vi "Count Up.vi"(7 "Reset":bool, 10 "Increment":bool) -> (2 "Count":i32)   [LabVIEW 2021]
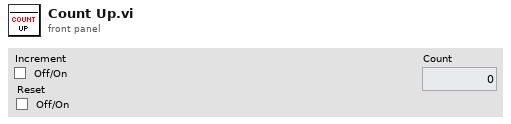
[diagram p1: front panel]
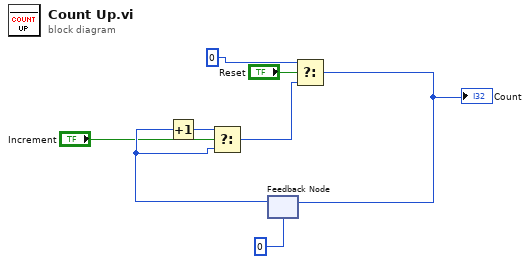
[diagram p0: block diagram]
diagram:
  n1 = feedback #1(0) -> (w6:i32)
  n2 = Increment(x=w6) -> (x+1=w5:i32)
  n3 = Select(t=w5, s="Increment", f=w6) -> (s? t:f=w4:i32)
  n4 = Select(t=0, s="Reset", f=w4) -> (s? t:f=w7:i32)
  "Count" <- w7
  n5 = feedback-in #1(w7) -> ()
